vi "TrajectoryCreateExecuteAbsolute.vi"(8 "Init":bool, 11 "End Pose ENG":T1={"TRANSLATION"={"X"=0.0, "Y"=0.0}, "ROTATION"={"VALUE"=0.0, "COS"=1.0, "SIN"=0.0}} {"ROTATION"."SIN" format="%13.4f"; "ROTATION"."COS" format="%13.4f"; "ROTATION"."VALUE" format="%13.4f"; "TRANSLATION"."Y" format="%14.3f"; "TRANSLATION"."X" format="%14.3f"}) -> (0 "AtReference":bool, 2 "Done":bool, 3 "Chassis Velocity Target":T4 {"vOmega" format="%10.3f"; "vY" format="%10.3f"; "vX" format="%10.3f"})   [LabVIEW 2023]
uses:
  <vilib>/Rock Robotics/WPI/ThirdParty/JAS_Junk/TrajLib/TypeDef/CHASSIS_SPEEDS.ctl
  <vilib>/Rock Robotics/WPI/ThirdParty/JAS_Junk/TrajLib/TypeDef/POSE2D.ctl
  <vilib>/Rock Robotics/WPI/ThirdParty/JAS_Junk/TrajLib/TypeDef/TRANSLATION2D.ctl
  <vilib>/Rock Robotics/WPI/ThirdParty/JAS_Junk/TrajLib/TypeDef/ROTATION2D.ctl
  <vilib>/Rock Robotics/WPI/ThirdParty/JAS_Junk/TrajLib/PIDController_Pack_Tuning.vi
  <vilib>/Rock Robotics/WPI/ThirdParty/JAS_Junk/TrajLib/HolDrvCtrl_PackProfPID.vi
  <vilib>/Rock Robotics/WPI/ThirdParty/JAS_Junk/TrajLib/VI/HolDrvCtrl_PackControllers.vi
  <vilib>/Rock Robotics/WPI/ThirdParty/JAS_Junk/TrajLib/Pose2d_New.vi
  <vilib>/Rock Robotics/WPI/ThirdParty/JAS_Junk/TrajLib/VI/Util_GetTime_U32.vi
  <vilib>/Rock Robotics/WPI/ThirdParty/JAS_Junk/TrajLib/HolDrvCtrl_New.vi
  <vilib>/Rock Robotics/WPI/ThirdParty/JAS_Junk/TrajLib/HolDrvCtrl_PackPID.vi
  <vilib>/Rock Robotics/WPI/ThirdParty/JAS_Junk/TrajLib/HolDrvCtrl_SetTolerance.vi
  <vilib>/Rock Robotics/WPI/ThirdParty/JAS_Junk/TrajLib/HolDrvCtrl_SetEnabled.vi
  <vilib>/Rock Robotics/WPI/ThirdParty/JAS_Junk/TrajLib/HolDrvCtrl_Calculate_Trajectory.vi
  <vilib>/Rock Robotics/WPI/ThirdParty/JAS_Junk/TrajLib/HolDrvCtrl_AtReference.vi
  <vilib>/Rock Robotics/WPI/ThirdParty/JAS_Junk/TrajLib/ProfiledPIDController_NewPeriod.vi
  <vilib>/Rock Robotics/WPI/ThirdParty/JAS_Junk/TrajLib/ProfiledPIDController_SetIntegratorRange.vi
  <vilib>/Rock Robotics/WPI/ThirdParty/JAS_Junk/TrajLib/ProfiledPIDController_DisableContInput.vi
  <vilib>/Rock Robotics/WPI/ThirdParty/JAS_Junk/TrajLib/ProfiledPIDController_EnableContInput.vi
  <vilib>/Rock Robotics/WPI/ThirdParty/JAS_Junk/TrajLib/TrapProfConstraint_New.vi
  <vilib>/Rock Robotics/WPI/ThirdParty/JAS_Junk/TrajLib/Rotation2d_CreateAngle.vi
  <vilib>/Rock Robotics/WPI/ThirdParty/JAS_Junk/TrajLib/Translation2d_Create.vi
  <vilib>/Rock Robotics/WPI/ThirdParty/JAS_Junk/TrajLib/Conv_Deg_Radians.vi
  <vilib>/Rock Robotics/WPI/ThirdParty/JAS_Junk/TrajLib/PIDController_NewPeriod.vi
  <vilib>/Rock Robotics/WPI/ThirdParty/JAS_Junk/TrajLib/PIDController_SetIntegratorRange.vi
  <vilib>/Rock Robotics/WPI/ThirdParty/JAS_Junk/TrajLib/PIDController_Reset.vi
  <vilib>/Rock Robotics/WPI/ThirdParty/JAS_Junk/TrajLib/HolDrvCtrl_Calculate.vi
  <vilib>/Rock Robotics/WPI/ThirdParty/JAS_Junk/TrajLib/Rotation2d_GetRadians.vi
  <vilib>/Rock Robotics/WPI/ThirdParty/JAS_Junk/TrajLib/TrapProfState_New.vi
  <vilib>/Rock Robotics/SystemInterfaces/NetworkCommunication/NetComm_UsageReport_report.vi
  <vilib>/Rock Robotics/WPI/ThirdParty/JAS_Junk/TrajLib/PIDController_DisableContinousInput.vi
  <vilib>/Rock Robotics/WPI/ThirdParty/JAS_Junk/TrajLib/PIDController_EnableContinousInput.vi
  <vilib>/Rock Robotics/WPI/ThirdParty/JAS_Junk/TrajLib/Rotation2d_GetAngleCosSin.vi
  <vilib>/Rock Robotics/WPI/ThirdParty/JAS_Junk/TrajLib/Pose2d_RelativeTo.vi
  <vilib>/Rock Robotics/WPI/ThirdParty/JAS_Junk/TrajLib/Pose2d_getRotation.vi
  <vilib>/Rock Robotics/WPI/ThirdParty/JAS_Junk/TrajLib/Rotation2d_Minus.vi
  <vilib>/Rock Robotics/WPI/ThirdParty/JAS_Junk/TrajLib/ProfiledPIDController_Calculate_Meas_Goal.vi
  <vilib>/Rock Robotics/WPI/ThirdParty/JAS_Junk/TrajLib/PIDController_Calculate_SP_PV.vi
  <vilib>/Rock Robotics/WPI/ThirdParty/JAS_Junk/TrajLib/ProfiledPIDController_Reset_PosOnly.vi
  <vilib>/Rock Robotics/WPI/ThirdParty/JAS_Junk/TrajLib/ChassisSpeeds_FromFieldRelativeSpeeds.vi
  <vilib>/Rock Robotics/WPI/ThirdParty/JAS_Junk/TrajLib/Transform2d_Create_PosePose.vi
  <vilib>/Rock Robotics/WPI/ThirdParty/JAS_Junk/TrajLib/Pose2d_New_TRRO.vi
  <vilib>/Rock Robotics/WPI/ThirdParty/JAS_Junk/TrajLib/Rotation2d_UnaryMinus.vi
  <vilib>/Rock Robotics/WPI/ThirdParty/JAS_Junk/TrajLib/Rotation2d_RotateBy.vi
  <vilib>/Rock Robotics/WPI/ThirdParty/JAS_Junk/TrajLib/ProfiledPIDController_SetGoal_PosOnly.vi
  <vilib>/Rock Robotics/WPI/ThirdParty/JAS_Junk/TrajLib/ProfiledPIDController_Calculate_Meas.vi
  <vilib>/Rock Robotics/WPI/ThirdParty/JAS_Junk/TrajLib/PIDController_SetSetpoint.vi
  <vilib>/Rock Robotics/WPI/ThirdParty/JAS_Junk/TrajLib/PIDController_Calculate_PV.vi
  <vilib>/Rock Robotics/WPI/ThirdParty/JAS_Junk/TrajLib/ProfiledPIDController_Reset.vi
  <vilib>/Rock Robotics/WPI/ThirdParty/JAS_Junk/TrajLib/Rotation2d_GetCos.vi
  <vilib>/Rock Robotics/WPI/ThirdParty/JAS_Junk/TrajLib/Rotation2d_GetSin.vi
  <vilib>/Rock Robotics/WPI/ThirdParty/JAS_Junk/TrajLib/Translation2d_RotateBy.vi
  <vilib>/Rock Robotics/WPI/ThirdParty/JAS_Junk/TrajLib/Translation2d_Minus.vi
  <vilib>/Rock Robotics/WPI/ThirdParty/JAS_Junk/TrajLib/Rotation2d_CreateXY.vi
  <vilib>/Rock Robotics/WPI/ThirdParty/JAS_Junk/TrajLib/ProfiledPIDController_SetGoal.vi
  <vilib>/Rock Robotics/WPI/ThirdParty/JAS_Junk/TrajLib/TrapProfile_New.vi
  <vilib>/Rock Robotics/WPI/ThirdParty/JAS_Junk/TrajLib/ProfiledPIDController_GetPeriod.vi
  <vilib>/Rock Robotics/WPI/ThirdParty/JAS_Junk/TrajLib/TrapProfile_Calculate.vi
  <vilib>/Rock Robotics/WPI/ThirdParty/JAS_Junk/TrajLib/ControllerUtil_GetModulusError.vi
  <vilib>/Rock Robotics/WPI/ThirdParty/JAS_Junk/TrajLib/Util_CalcDist.vi
  <vilib>/Rock Robotics/WPI/ThirdParty/JAS_Junk/TrajLib/TrapProfile_ShouldFlipAcceleration.vi
  <vilib>/Rock Robotics/WPI/ThirdParty/JAS_Junk/TrajLib/TrapProfile_Direct.vi
  <vilib>/Rock Robotics/WPI/ThirdParty/JAS_Junk/TrajLib/PIDController_GetPeriod.vi
  <vilib>/Rock Robotics/WPI/ThirdParty/JAS_Junk/TrajLib/VI/Util_GetTime_U64.vi
  TrajectoryGlobals.vi
  Vision/VisionGlobal.vi
  <vilib>/Rock Robotics/WPI/ThirdParty/JAS_Junk/TrajLib/Globals/Util_LibraryGlobals.vi
  Drive/DriveGlobal.vi
  <vilib>/Rock Robotics/WPI/ThirdParty/JAS_Junk/TrajLib/Trajectory_Library.lvlib
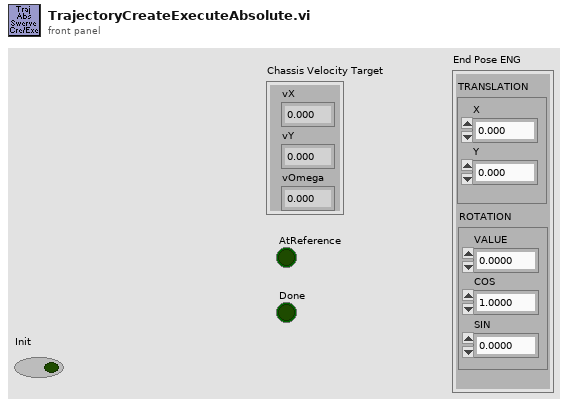
[diagram p1: front panel]
types:
  T1 = typedef "Trajectory_Library.lvlib/POSE2D.ctl" = cluster{"TRANSLATION":T2, "ROTATION":T3}
  T2 = typedef "Trajectory_Library.lvlib/TRANSLATION2D.ctl" = cluster{"X":dbl, "Y":dbl}
  T3 = typedef "Trajectory_Library.lvlib/ROTATION2D.ctl" = cluster{"VALUE":dbl, "COS":dbl, "SIN":dbl}
  T4 = typedef "Trajectory_Library.lvlib/CHASSIS_SPEEDS.ctl" = cluster{"vX":dbl, "vY":dbl, "vOmega":dbl}
  T5 = typedef "Trajectory_Library.lvlib/SWERVE_DRIVE_KINEMATICS.ctl" = cluster{"NumModules":i32, "InverseKinematics":T6, "ForwardKinematics":T6, "Modules":T2[], "PrevCoR":T2, "SavedModuleStates":T7[]}
  T6 = typedef "NI_Matrix.lvlib/RealMatrix.ctl" = dbl[][]
  T7 = typedef "Trajectory_Library.lvlib/SWERVE_DRIVE_MODULE_STATE.ctl" = cluster{"Speed":dbl, "Angle":T3}
  T8 = typedef "Trajectory_Library.lvlib/TRAJECTORY.ctl" = cluster{"TotalTImeSecs":dbl, "States":T9[]}
  T9 = typedef "Trajectory_Library.lvlib/TRAJ_STATE.ctl" = cluster{"TimeSeconds":dbl, "Velocity":dbl, "Acceleration":dbl, "POSE":T1, "Curvature":dbl}
  T10 = typedef "Trajectory_Library.lvlib/HOLONOMIC_PACK_TUNING.ctl" = cluster{"X PID Tuning":T11, "Y PID Tuning":T11, "thetaProfiledPID_CTRL":T12}
  T11 = typedef "Trajectory_Library.lvlib/PID_TUNING.ctl" = cluster{"Kp":dbl, "Ki":dbl, "Kd":dbl, "MaximumIntegral":dbl, "MinimumIntegral":dbl, "IntegralZone":dbl}
  T12 = typedef "Trajectory_Library.lvlib/PROFILED_PID_CONTROLLER.ctl" = cluster{"Controller":T13, "Goal":T14, "Setpoint":T14, "Constraint":T15}
  T13 = typedef "Trajectory_Library.lvlib/PID_CONTROLLER.ctl" = cluster{"Kp":dbl, "Ki":dbl, "Kd":dbl, "Period":dbl, "Max_Integral":dbl, "Min_Integral":dbl, "Max_Input":dbl, "Min_Input":dbl, "Continuous":bool, "PositionError":dbl, "VelocityError":dbl, "PrevError":dbl, "Total_Integral":dbl, "PositionTolerance":dbl, "VelocityTolerance":dbl, "SetPoint":dbl, "Kf":dbl, "Prev_Deriv":dbl, "Prev_Deriv 2":dbl, "DerivativeFilter":bool, "Min_Output":dbl, "Max_Output":dbl, "Prev_F_P":dbl, "Prev_F_P_2":dbl, "AntiWindupActive":bool, "Measurement":dbl, "IntegralZone":dbl}
  T14 = typedef "Trajectory_Library.lvlib/TRAPEZOID_PROFILE_STATE.ctl" = cluster{"Position":dbl, "Velocity":dbl}
  T15 = typedef "Trajectory_Library.lvlib/TRAPEZOID_PROFILE_CONSTRAINT.ctl" = cluster{"MaxVelocity":dbl, "MaxAcceleration":dbl}
  T16 = typedef "Trajectory_Library.lvlib/HOLONOMIC_DRV_CTRL.ctl" = cluster{"poseTolerance":T1, "poseError":T1, "Enabled":bool, "PID_xCtrl":T13, "PID_yCtrl":T13, "PROF_PID_thetaCtrl":T12, "RotationError":T3, "FirstRun":bool}
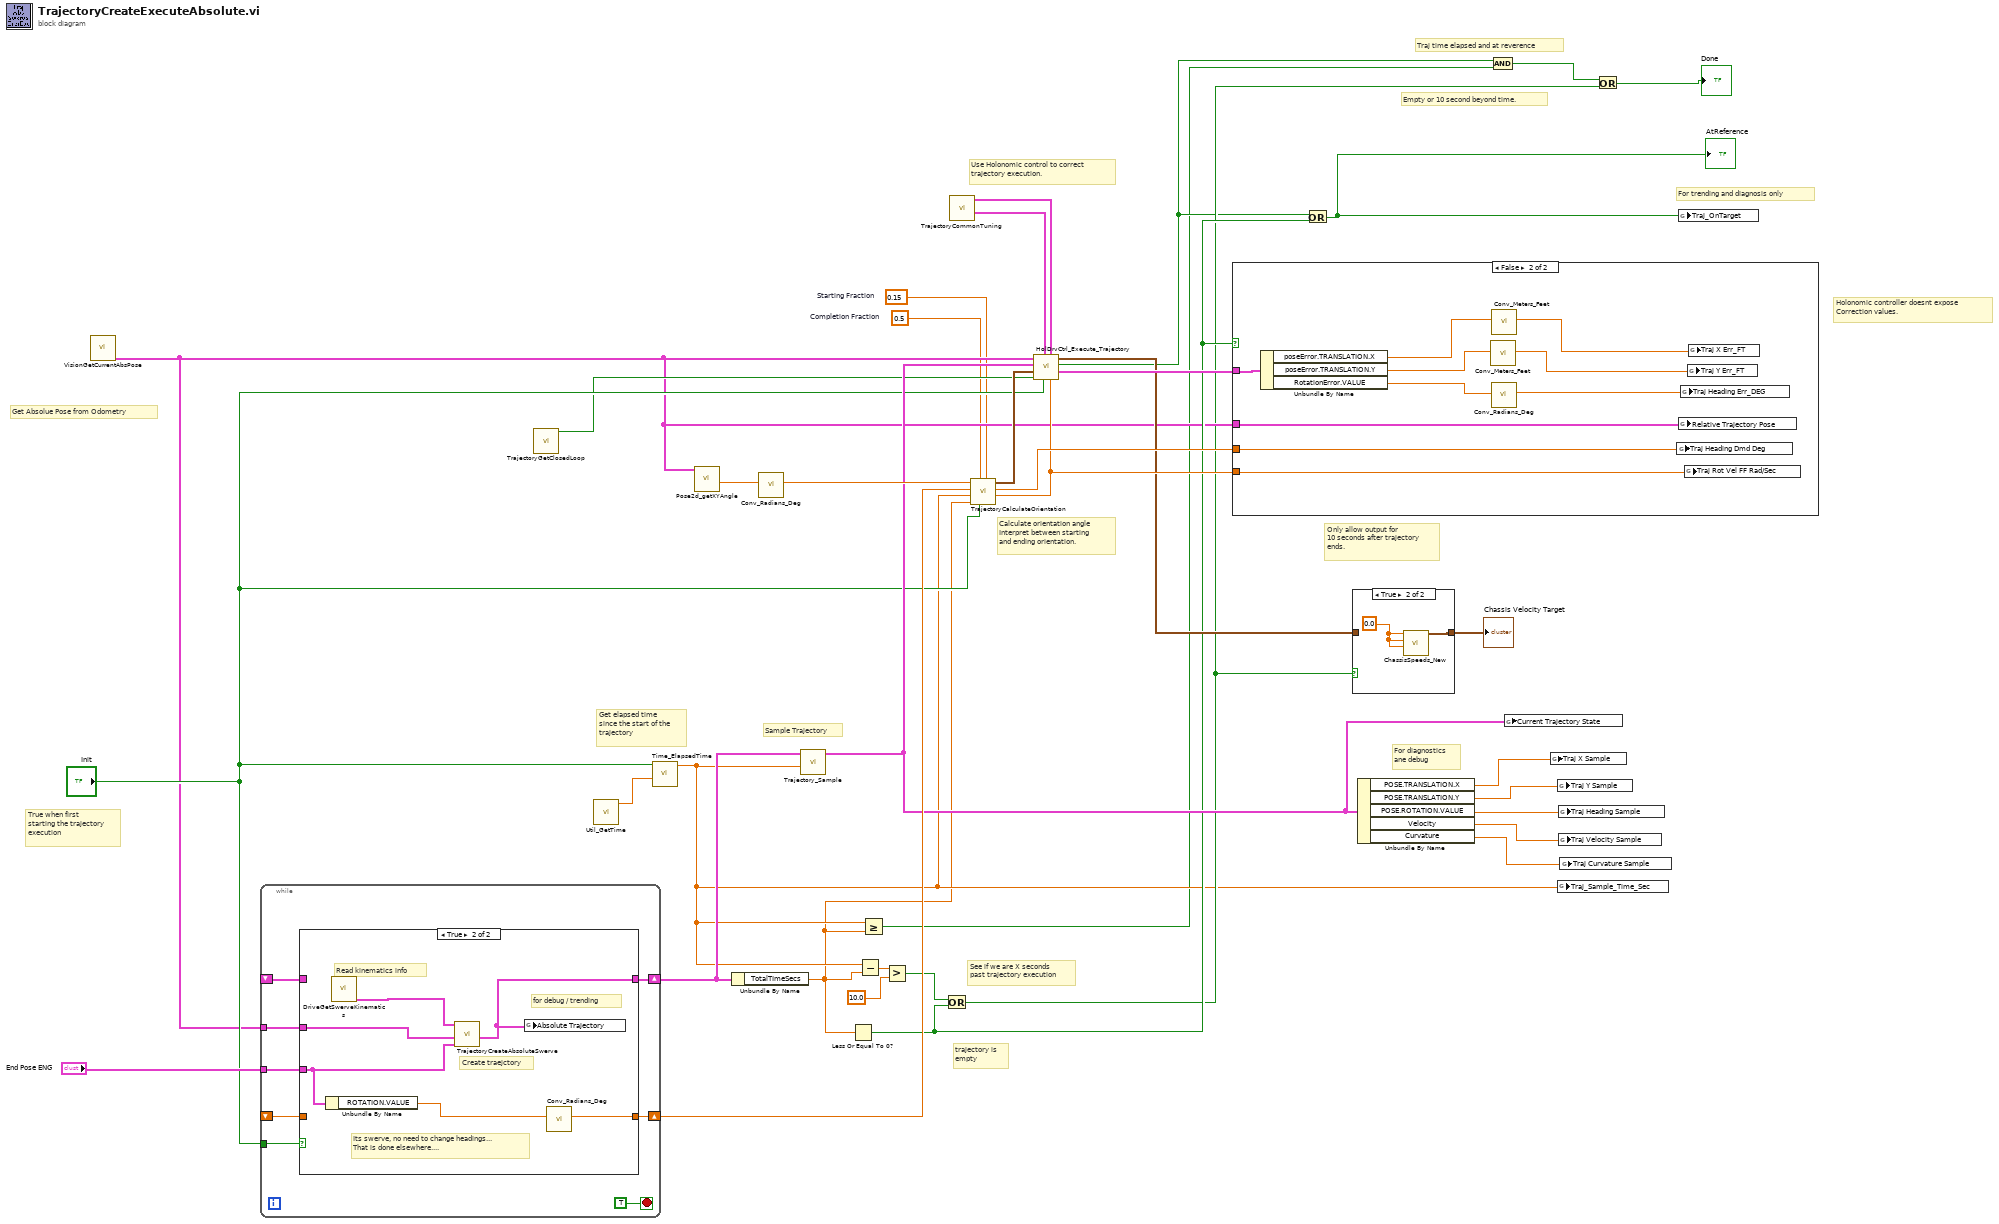
[diagram p0: block diagram]
diagram:
  w10 = 0.5  # Completion Fraction
  w11 = 0.15  # Starting Fraction
  # "Traj time elapsed and at reverence"
  # "Empty or 10 second beyond time."
  # "trajectory is \nempty"
  # "Calculate orientation angle\nInterpret between starting\nand ending orientation."
  # "True when first\nstarting the trajectory\nexecution"
  # "Get elapsed time\nsince the start of the\ntrajectory"
  # "Holonomic controller doesnt expose\nCorrection values."
  # "Use Holonomic control to correct\ntrajectory execution."
  # "For trending and diagnosis only"
  # "For diagnostics\nane debug"
  # "Get Absolue Pose from Odometry"
  # "Sample Trajectory"
  # "See if we are X seconds \npast trajectory execution"
  # "Only allow output for\n10 seconds after trajectory\nends."
  n1 = call "VisionGetCurrentAbsPose.vi"() -> ("Current ABS Pose"=w12:T1)  [unwired: 9 in]
  n2 = while {
    tunnel: "Init" -> [w44]
    tunnel: w12 -> [w43]
    shift-right: [w42] -> w24
    shift-left: _ -> [w41]
    shift-right: [w40] -> w21
    shift-left: _ -> [w39]
    tunnel: "End Pose ENG" -> [w38]
    stop <- TRUE stop-if-true
    n3 = case shown="True" w44 {
      tunnel: w43 -> [_ w49]
      tunnel: [w47 w50] -> w42
      tunnel: w41 -> [w47 _]
      tunnel: [w46 w52] -> w40
      tunnel: w39 -> [w46 _]
      tunnel: w38 -> [_ w53]
      frame False {
      }
      frame True {
        # "for debug / trending"
        # "Read kinematics info"
        # "Its swerve, no need to change headings...\nThat is done elsewhere...."
        # "Create traejctory"
        n4 = Unbundle By Name(w53) -> ("ROTATION.VALUE"=w51:dbl)
        n5 = call "DriveGetSwerveKinematics.vi"() -> ("SWERVE_DRIVE_KINEMATICS"=w48:T5)  [unwired: 11 in]
        n6 = call "TrajectoryCreateAbsoluteSwerve.vi"("End Pose  ENG"=w53, "Current Pose SI"=w49, "SWERVE_DRIVE_KINEMATICS"=w48) -> ("Absolute Trajectory"=w50:T8)  [unwired: 6 in, 2 out]
        n7 = global write "TrajectoryGlobals.vi" "Absolute Trajectory"(w50) -> ()
        n8 = call <vilib>:"Conv_Radians_Deg.vi"("Radians"=w51) -> ("Degrees"=w52:dbl)  [unwired: 10 in]
      }
    }
  }
  n9 = call "TrajectoryGetClosedLoop.vi"() -> ("AUTO_CLOSED_LOOP"=w13:bool)  [unwired: 11 in]
  n10 = call <vilib>:"Util_GetTime.vi"() -> ("FPGA_Time_Seconds"=w34:dbl)  [unwired: 9 in, 2 out]
  n11 = call <vilib>:"Time_ElapsedTime.vi"("PassthroughTime_SEC"=w34, "Reset"="Init") -> ("Elapsed Time Sec"=w3:dbl)  [unwired: 9 in]
  n12 = call <vilib>:"Pose2d_getXYAngle.vi"("in POSE"=w12) -> ("Angle"=w23:dbl)  [unwired: 8 in, 2 out]
  n13 = Unbundle By Name(w24) -> ("TotalTImeSecs"=w2:dbl)
  n14 = call <vilib>:"Conv_Radians_Deg.vi"("Radians"=w23) -> ("Degrees"=w22:dbl)  [unwired: 10 in]
  n15 = call <vilib>:"Trajectory_Sample.vi"("Time"=w3, "InputTRAJECTORY"=w24) -> ("OutputTRAJ_STATE"=w20:T9)  [unwired: 9 in]
  n16 = Less Or Equal To 0?(x=w2) -> (x <= 0?=w15:bool)
  n17 = Subtract(x=w3, y=w2) -> (x-y=w37:dbl)
  n18 = Greater Or Equal?(x=w3, y=w2) -> (x >= y?=w1:bool)
  n19 = Greater?(x=w37, y=10.0) -> (0:w17:bool)
  n20 = Or(x=w17, y=w15) -> (x .or. y?=w5:bool)
  n21 = call "TrajectoryCommonTuning.vi"() -> ("out POSe"=w8:T1, "HOLONOMIC_CTRL_PACK_TUNING"=w9:T10)  [unwired: 10 in]
  n22 = call "TrajectoryCalculateOrientation.vi"("Starting Fraction"=w11, "Init"="Init", "Completion Fraction"=w10, "Total Trajectory Time Sec"=w2, "Elapsed Traj Time Sec"=w3, "End Orientation Demand DEG"=w21, "Starting Orientation  DEG"=w22) -> ("Rotational Velocity Rad Per Sec"=w25:dbl, "Orientation Demand Deg"=w28:dbl, "Orientation Demand"=w27:T3)  [unwired: 2 in]
  n23 = call <vilib>:"HolDrvCtrl_Execute_Trajectory.vi"("Rotational Velocity Feedforward \nRad/Sec"=w25, "HOLONOMIC_CTRL_PACK_TUNING"=w9, "Reset"="Init", "Tolerance"=w8, "Enable"=w13, "angleRef"=w27, "desiredTrajState"=w20, "currentPose"=w12) -> ("outHOLONOMIC_DRV_CTRL"=w26:T16, "AtReference"=w4:bool, "calcChassisSpeed"=w18:T4)  [unwired: 1 in]
  n24 = case shown="False" w15 {
    tunnel: w28 -> [_ w63]
    tunnel: w26 -> [_ w57]
    tunnel: w25 -> [_ w56]
    tunnel: w12 -> [_ w54]
    frame True {
    }
    frame False {
      n25 = Unbundle By Name(w57) -> ("poseError.TRANSLATION.X"=w61:dbl, "poseError.TRANSLATION.Y"=w60:dbl, "RotationError.VALUE"=w55:dbl)
      n26 = call <vilib>:"Conv_Meters_Feet.vi"("Meters"=w60) -> ("Feet"=w59:dbl)  [unwired: 10 in]
      n27 = call <vilib>:"Conv_Radians_Deg.vi"("Radians"=w55) -> ("Degrees"=w62:dbl)  [unwired: 10 in]
      n28 = call <vilib>:"Conv_Meters_Feet.vi"("Meters"=w61) -> ("Feet"=w58:dbl)  [unwired: 10 in]
      n29 = global write "TrajectoryGlobals.vi" "Traj Heading Dmd Deg"(w63) -> ()
      n30 = global write "TrajectoryGlobals.vi" "Relative Trajectory Pose"(w54) -> ()
      n31 = global write "TrajectoryGlobals.vi" "Traj Heading Err_DEG"(w62) -> ()
      n32 = global write "TrajectoryGlobals.vi" "Traj Rot Vel FF Rad/Sec"(w56) -> ()
      n33 = global write "TrajectoryGlobals.vi" "Traj Y Err_FT"(w59) -> ()
      n34 = global write "TrajectoryGlobals.vi" "Traj X Err_FT"(w58) -> ()
    }
  }
  n35 = Or(x=w4, y=w15) -> (x .or. y?=w16:bool)
  "AtReference" <- w16
  n36 = case shown="True" w5 {
    tunnel: w18 -> [w64 _]
    tunnel: [w64 w65] -> w35
    frame False {
    }
    frame True {
      w66 = 0.0 ("vX")
      n37 = call <vilib>:"ChassisSpeeds_New.vi"("vAngular"=w66, "vY"=w66, "vX"=w66) -> ("CHASSIS"=w65:T4)  [unwired: 8 in]
    }
  }
  "Chassis Velocity Target" <- w35
  n38 = Unbundle By Name(w20) -> ("POSE.TRANSLATION.X"=w33:dbl, "POSE.TRANSLATION.Y"=w32:dbl, "POSE.ROTATION.VALUE"=w31:dbl, "Velocity"=w30:dbl, "Curvature"=w29:dbl)
  n39 = And(x=w4, y=w1) -> (x .and. y?=w6:bool)
  n40 = global write "TrajectoryGlobals.vi" "Current Trajectory State"(w20) -> ()
  n41 = global write "TrajectoryGlobals.vi" "Traj X Sample"(w33) -> ()
  n42 = global write "TrajectoryGlobals.vi" "Traj Y Sample"(w32) -> ()
  n43 = global write "TrajectoryGlobals.vi" "Traj_Sample_Time_Sec"(w3) -> ()
  n44 = global write "TrajectoryGlobals.vi" "Traj Heading Sample"(w31) -> ()
  n45 = global write "TrajectoryGlobals.vi" "Traj Velocity Sample"(w30) -> ()
  n46 = global write "TrajectoryGlobals.vi" "Traj Curvature Sample"(w29) -> ()
  n47 = Or(x=w6, y=w5) -> (x .or. y?=→"Done":bool)
  n48 = global write "TrajectoryGlobals.vi" "Traj_OnTarget"(w16) -> ()
